vi "AlliGator Set Phasor Ratio Display Range.vi"(8 "error in (no error)":errorcluster, 11 "Phasor Ratio Display Range":refnum<vi>) -> (0 "error out":errorcluster)   [LabVIEW 2021, in "AlliGator Settings.lvlib"]
doc: "Constrains the sliders of the Phasor Ratio (or other parameter) Range to the displayed slide's min and max values."
uses:
  AlliGator Settings.lvlib
panel:
  # "see the AlliGator License on the block diagram (Ctrl+E or Window:Show Block Diagram)"
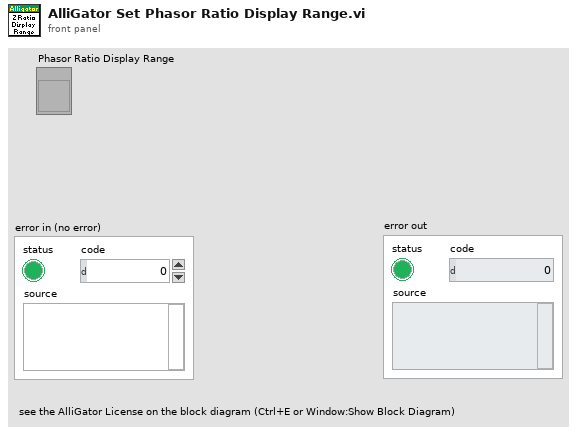
[diagram p1: front panel]
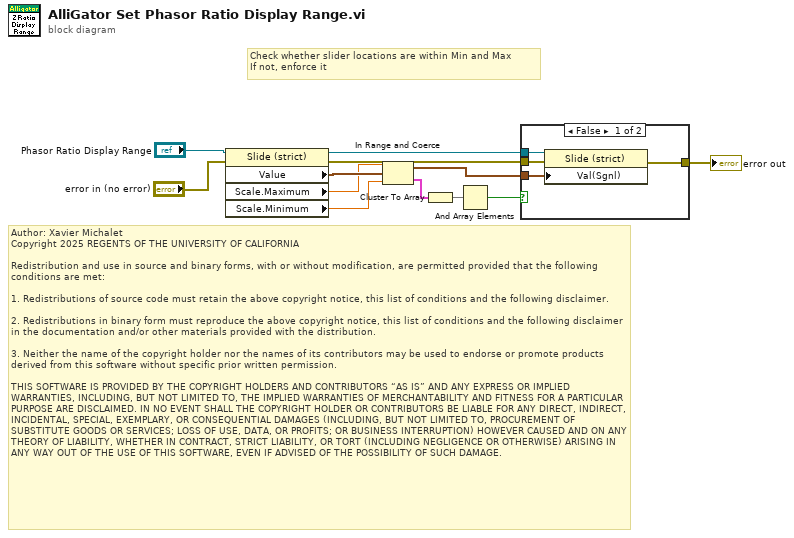
[diagram p0: block diagram]
diagram:
  # "Author: Xavier Michalet\nCopyright 2025 REGENTS OF THE UNIVERSITY OF CALIFORNIA\n\nRedistribution and use in source and binary forms, with or without modification, are permitted provided that the following conditions are met:\n\n1. Redistributions of source code must retain the above copyright notice, this list of conditions and the following disclaimer.\n\n2. Redistributions in binary form must reproduce the above copyright notice, this list of conditions and the following disclaimer in the documentation and/or other materials provided with the distribution.\n\n3. Neither the name of the copyright holder nor the names of its contributors may be used to endorse or promote products derived from this software without specific prior written permission.\n\nTHIS SOFTWARE IS PROVIDED BY THE COPYRIGHT HOLDERS AND CONTRIBUTORS “AS IS” AND ANY EXPRESS OR IMPLIED WARRANTIES, INCLUDING, BUT NOT LIMITED TO, THE IMPLIED WARRANTIES OF MERCHANTABILITY AND FITNESS FOR A PARTICULAR PURPOSE ARE DISCLAIMED. IN NO EVENT SHALL THE COPYRIGHT HOLDER OR CONTRIBUTORS BE LIABLE FOR ANY DIRECT, INDIRECT, INCIDENTAL, SPECIAL, EXEMPLARY, OR CONSEQUENTIAL DAMAGES (INCLUDING, BUT NOT LIMITED TO, PROCUREMENT OF SUBSTITUTE GOODS OR SERVICES; LOSS OF USE, DATA, OR PROFITS; OR BUSINESS INTERRUPTION) HOWEVER CAUSED AND ON ANY THEORY OF LIABILITY, WHETHER IN CONTRACT, STRICT LIABILITY, OR TORT (INCLUDING NEGLIGENCE OR OTHERWISE) ARISING IN ANY WAY OUT OF THE USE OF THIS SOFTWARE, EVEN IF ADVISED OF THE POSSIBILITY OF SUCH DAMAGE."
  # "Check whether slider locations are within Min and Max\nIf not, enforce it"
  n1 = property class="Slide (strict)"(reference="Phasor Ratio Display Range", error in="error in (no error)") -> (reference out=w3:refnum<vi>, error out=w2:errorcluster, "Value"=w10:cluster{dbl, dbl}, "Scale.Maximum"=w9:dbl, "Scale.Minimum"=w8:dbl)
  n2 = In Range and Coerce(upper limit=w9, x=w10, lower limit=w8) -> (coerced(x)=w7:cluster{dbl, dbl}, In Range?=w6:cluster{bool, bool})
  n3 = Cluster To Array(cluster=w6) -> (array=w5:bool[])
  n4 = And Array Elements(Boolean array=w5) -> (logical AND=w4:bool)
  n5 = case shown="False" w4 {
    tunnel: w7 -> [w16 _]
    tunnel: w3 -> [w15 _]
    tunnel: w2 -> [w14 w17]
    tunnel: [w13 w17] -> w1
    frame False {
      n6 = property class="Slide (strict)"(reference=w15, error in=w14, "Val(Sgnl)"=w16) -> (error out=w13:errorcluster)  [unwired: 1 out]
    }
    frame True {
    }
  }
  "error out" <- w1
